vi "ShutterInitialize.vi"(8 "error in (no error)":errorcluster, 11 "Microscope in":refnum<class "Microscope.lvclass">) -> (0 "error out":errorcluster, 3 "Microscope out":refnum<class "Microscope.lvclass">)   [LabVIEW 2012, in "Microscope.lvclass"]
doc: "Loads all shutters and closes them."
uses:
  classes/Microscope.lvclass
  classes/Microscope.lvclass/Microscope.ctl
  <vilib>/DAQmx/write.llb/DAQmx Write (Digital Bool 1Line 1Point).vi
  <vilib>/DAQmx/create/channels.llb/DAQmx Create Channel (DO-Digital Output).vi
  <vilib>/DAQmx/miscellaneous.llb/DAQmx Fill In Error Info.vi
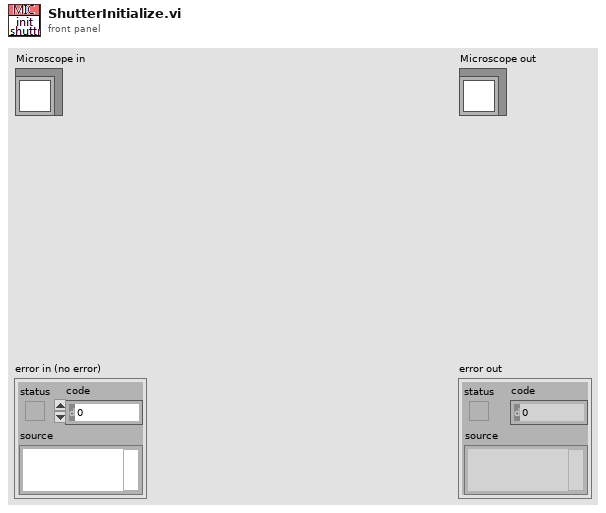
[diagram p1: front panel]
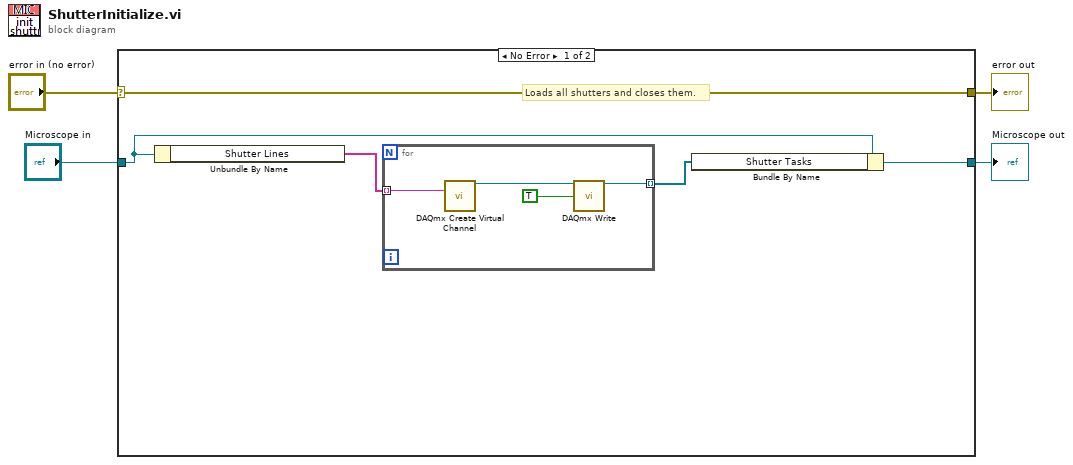
[diagram p0: block diagram]
diagram:
  n1 = case shown="No Error" "error in (no error)" {
    selector: "error in (no error)" -> [w9 w15]
    tunnel: [w9 w15] -> w3
    tunnel: [w6 w14] -> w1
    tunnel: "Microscope in" -> [w7 w14]
    frame No Error {
      # "Loads all shutters and closes them."
      n2 = Unbundle By Name(w7) -> ("Shutter Lines"=w8:tag[])
      n3 = for {
        tunnel: w8 -> [w13] mode=indexing
        tunnel: [w10] -> w5 mode=indexing
        n4 = call-poly <vilib>:"DAQmx Create Virtual Channel.vi"("lines"=w13) -> ("task out"=w11:refnum<k21>)  [unwired: 13 in, 1 out]
        n5 = call-poly <vilib>:"DAQmx Write.vi"("task/channels in"=w11, "data"=TRUE) -> ("task out"=w10:refnum<k21>)  [unwired: 11 in, 2 out]
      }
      n6 = Bundle By Name(cluster=w7, "Shutter Tasks"=w5) -> (w6:refnum<class "Microscope.lvclass">)
    }
    frame Error {
    }
  }
  "error out" <- w3
  "Microscope out" <- w1
